vi "Launcher.vi"   [LabVIEW 2020, in "GUI.lvlib"]
uses:
  GUI.lvlib
  GUI.lvclass
  C:/Program Files/National Instruments/LabVIEW 2020/vi.lib/ActorFramework/Actor/Actor.lvclass
  <vilib>/ActorFramework/Actor/Actor.lvclass
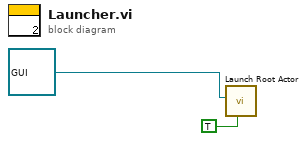
[diagram p0: block diagram]
diagram:
  n1 = call <vilib>:"Launch Root Actor.vi"("Open Actor Core front panel? (F)"=TRUE, "Actor"=refnum<class "GUI.lvclass"> refnum ("GUI.lvlib:GUI.lvclass")) -> ()  [unwired: 8 in, 2 out]
